vi "traces_close_sub.vi"(8 "error in (no error)":errorcluster, 10 "traces":cluster{"idx":u32}[](array[cluster]), 11 "traces used":u64) -> (0 "error out":errorcluster, 3 "traces used out":u64)   [LabVIEW 2010, in "OSA.lvclass"]
uses:
  OSA.lvclass
  FTSLib.dll
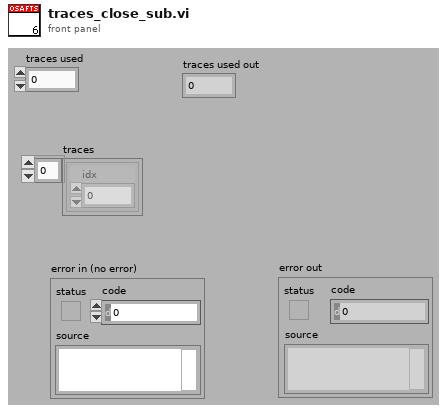
[diagram p1: front panel]
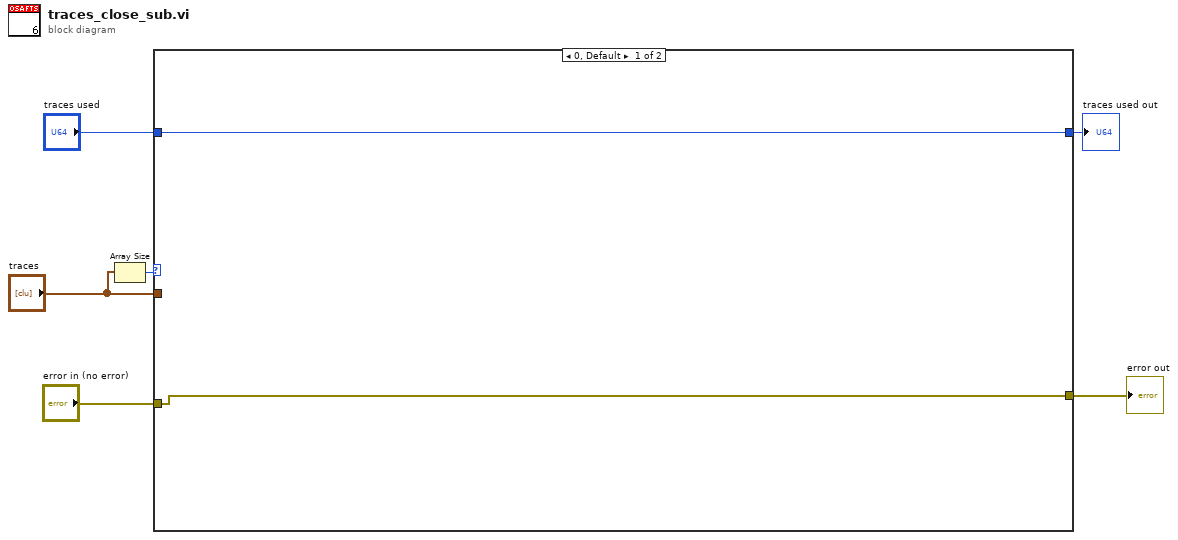
[diagram p0: block diagram]
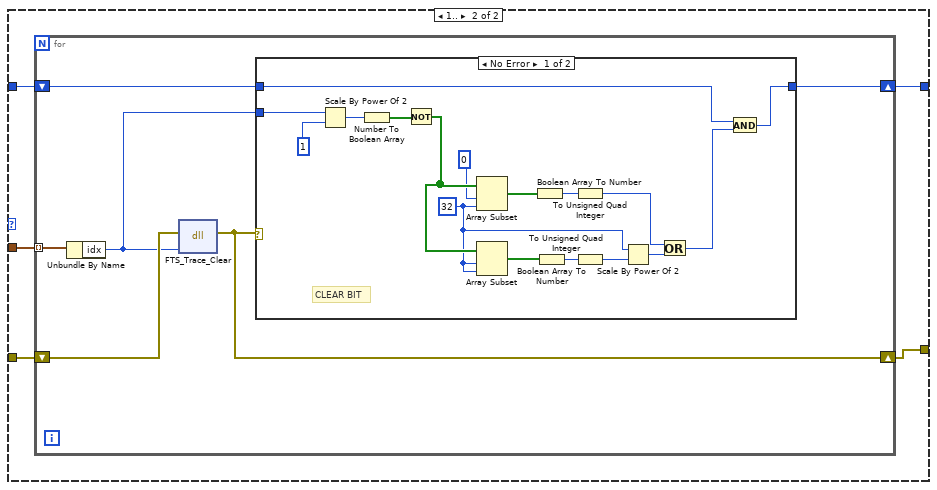
[diagram p2: hidden frame]
diagram:
  n1 = Array Size(array="traces") -> (size(s)=w6:i32)
  n2 = case shown="0, Default" w6 {
    tunnel: "traces" -> [_ w13]
    tunnel: "error in (no error)" -> [w7 w12]
    tunnel: "traces used" -> [w8 w11]
    tunnel: [w8 w10] -> w3
    tunnel: [w7 w9] -> w1
    frame 0, Default {
    }
    frame 1.. {
      n3 = for {
        tunnel: w13 -> [w19] mode=indexing
        shift-right: [w14] -> w9
        shift-left: w12 -> [w18]
        shift-right: [w15] -> w10
        shift-left: w11 -> [w17]
        n4 = Unbundle By Name(w19) -> ("idx"=w16:u32)
        n5 = dll-call lib="FTSLib.dll" fn="FTS_Trace_Clear"(error in=w18, "idx_buffer"=w16) -> (error out=w14:errorcluster)  [unwired: 4 in, 1 out]
        n6 = case shown="No Error" w14 {
          tunnel: w17 -> [w23 w37]
          tunnel: w16 -> [w22 _]
          tunnel: [w20 w37] -> w15
          frame No Error {
            w26 = 32 ("length")
            # "CLEAR BIT"
            n7 = Scale By Power Of 2(n=w22, x=u64 1) -> (x*2^n=w35:u64)
            n8 = Number To Boolean Array(number=w35) -> (Boolean array=w34:bool[])
            n9 = Not(x=w34) -> (.not. x?=w33:bool[])
            n10 = Array Subset(array=w33, index=0, length=w26) -> (w30:bool[])
            n11 = Array Subset(array=w33, index=w26, length=w26) -> (w31:bool[])
            n12 = Boolean Array To Number(Boolean array=w30) -> (number=w28:u32)
            n13 = Boolean Array To Number(Boolean array=w31) -> (number=w29:u32)
            n14 = To Unsigned Quad Integer(1:w28) -> (0:w24:u64)
            n15 = To Unsigned Quad Integer(1:w29) -> (0:w27:u64)
            n16 = Scale By Power Of 2(n=w26, x=w27) -> (x*2^n=w25:u64)
            n17 = Or(x=w24, y=w25) -> (x .or. y?=w21:u64)
            n18 = And(x=w23, y=w21) -> (x .and. y?=w20:u64)
          }
          frame Error {
          }
        }
      }
    }
  }
  "traces used out" <- w3
  "error out" <- w1
